vi "Get Strings from Enum__csm.vi"(8 "error in (no error)":errorcluster, 10 "Enum":variant) -> (0 "error out":errorcluster, 1 "String Value":string, 2 "Enum Strings":string[](array[string]), 3 "Enum Name":string)   [LabVIEW 2017, in "API String Arguments Support.lvlib"]
doc: "Returns Enum Strings array, String Value and Enum Name from an Enum."
uses:
  API String Arguments Support.lvlib
  <userlib>/_NEVSTOP/Communicable State Machine(CSM)/Communicable State Machine.lvlib
panel:
  # "[OpenG VI Tags] ***Do Not Remove***"
  # "Get Strings from Enum.vi\n\nReturns Enum Strings array, String Value and Enum Name from an Enum.\n\nPlease visit http://www.OpenG.org to learn about the\nOpen Source LabVIEW software movement.\n\nNOTICE -- YOU MUST LEAVE THIS NOTICE IN PLACE.  PER THE TERMS OF THE LICENSE BELOW, YOU MAY SUBLICENSE THIS SOFTWARE \nIN ANY WAY THAT DOES NOT CONFLICT WITH THIS LICENSE.\n\n### BSD License (http://www.opensource.org/licenses/bsd-license.php) Begin ###\n \nCopyright (c) 2002, Jean-Pierre Drolet <drolet_jp@hotmail.com>\nCopyright (c) 2002-2006, Jim Kring <jim@jimkring.com>\n\nAll rights reserved.\n\nRedistribution and use in source and binary forms, with or without modification, are permitted provided that the following conditions are met:\n\n    * Redistributions of source code must retain the above copyright notice, this list of conditions and the following disclaimer.\n    * Redistributions in binary form must reproduce the above copyright notice, this list of conditions and the following disclaimer in the \n       documentation and/or other materials provided with the distribution.\n    * Neither the name of SciWare, James Kring, Inc., nor the names of its contributors may be used to endorse or promote products derived \n       from this software without specific prior written permission.\n\nTHIS SOFTWARE IS PROVIDED BY THE COPYRIGHT HOLDERS AND CONTRIBUTORS \"AS IS\" AND ANY EXPRESS OR IMPLIED WARRANTIES, \nINCLUDING, BUT NOT LIMITED TO, THE IMPLIED WARRANTIES OF MERCHANTABILITY AND FITNESS FOR A PARTICULAR PURPOSE ARE \nDISCLAIMED. IN NO EVENT SHALL THE COPYRIGHT OWNER OR CONTRIBUTORS BE LIABLE FOR ANY DIRECT, INDIRECT, INCIDENTAL,\n SPECIAL, EXEMPLARY, OR CONSEQUENTIAL DAMAGES (INCLUDING, BUT NOT LIMITED TO, PROCUREMENT OF SUBSTITUTE GOODS OR \nSERVICES; LOSS OF USE, DATA, OR PROFITS; OR BUSINESS INTERRUPTION) HOWEVER CAUSED AND ON ANY THEORY OF LIABILITY, \nWHETHER IN CONTRACT, STRICT LIABILITY, OR TORT (INCLUDING NEGLIGENCE OR OTHERWISE) ARISING IN ANY WAY OUT OF THE USE \nOF THIS SOFTWARE, EVEN IF ADVISED OF THE POSSIBILITY OF SUCH DAMAGE.\n\n### BSD License End ###"
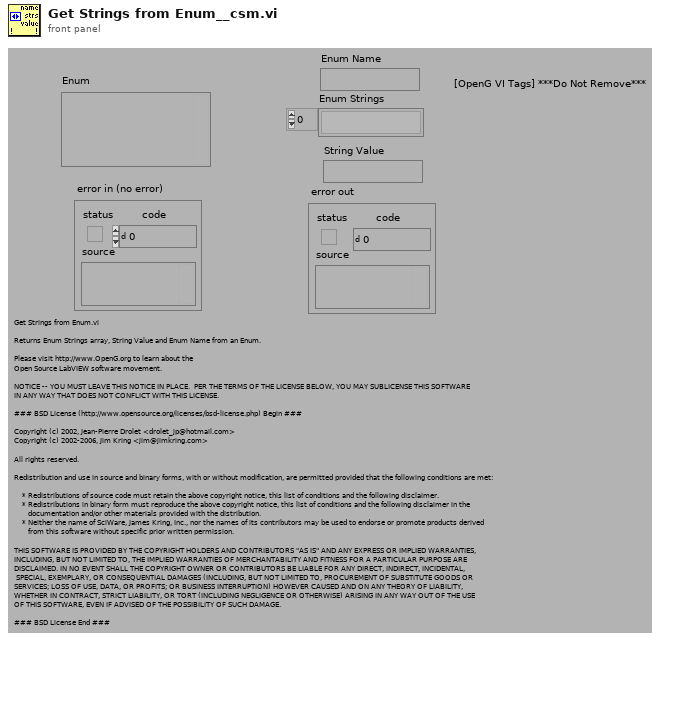
[diagram p1: front panel]
types:
  T1 = cluster{"length":u16, "private":u8, "type":enum8{"<Null>", "I8", "I16", "I32", "I64", "U8", "U16", "U32", "U64", "SGL", "DBL", "EXT", "CSG", "CDB", "CXT", "0x0F", "0x10", "0x11", "0x12", "0x13", "0x14", "Enum U8", "Enum U16", "Enum U32", "Enum U64", "SGL PQ", "DBL PQ", "EXT PQ", "CSG PQ", "CDB PQ", "CXT PQ", "0x1F", "0x20", "Boolean", "0x22", "0x23", "0x24", "0x25", "0x26", "0x27", "0x28", "0x29", "0x2A", "0x2B", "0x2C", "0x2D", "0x2E", "0x2F", "String", "0x31", "Path", "Pict", "0x34", "0x35", "0x36", "DAQ", "0x38", "0x39", "0x3A", "0x3B", "0x3C", "0x3D", "0x3E", "0x3F", "Array", "0x41", "0x42", "0x43", "0x44", "0x45", "0x46", "0x47", "0x48", "0x49", "0x4A", "0x4B", "0x4C", "0x4D", "0x4E", "0x4F", "Cluster", "0x51", "0x52", "Variant", "Waveform", "0x55", "0x56", "0x57", "0x58", "0x59", "0x5A", "0x5B", "0x5C", "0x5D", "0x5E", "Fixed Point", "0x60", "0x61", "0x62", "0x63", "0x64", "0x65", "0x66", "0x67", "0x68", "0x69", "0x6A", "0x6B", "0x6C", "0x6D", "0x6E", "0x6F", "Refnum", "0x71", "0x72", "Set Collection", "Map Collection"}, "# elements":u16}
  T2 = enum8{"<Null>", "I8", "I16", "I32", "I64", "U8", "U16", "U32", "U64", "SGL", "DBL", "EXT", "CSG", "CDB", "CXT", "0x0F", "0x10", "0x11", "0x12", "0x13", "0x14", "Enum U8", "Enum U16", "Enum U32", "Enum U64", "SGL PQ", "DBL PQ", "EXT PQ", "CSG PQ", "CDB PQ", "CXT PQ", "0x1F", "0x20", "Boolean", "0x22", "0x23", "0x24", "0x25", "0x26", "0x27", "0x28", "0x29", "0x2A", "0x2B", "0x2C", "0x2D", "0x2E", "0x2F", "String", "0x31", "Path", "Pict", "0x34", "0x35", "0x36", "DAQ", "0x38", "0x39", "0x3A", "0x3B", "0x3C", "0x3D", "0x3E", "0x3F", "Array", "0x41", "0x42", "0x43", "0x44", "0x45", "0x46", "0x47", "0x48", "0x49", "0x4A", "0x4B", "0x4C", "0x4D", "0x4E", "0x4F", "Cluster", "0x51", "0x52", "Variant", "Waveform", "0x55", "0x56", "0x57", "0x58", "0x59", "0x5A", "0x5B", "0x5C", "0x5D", "0x5E", "Fixed Point", "0x60", "0x61", "0x62", "0x63", "0x64", "0x65", "0x66", "0x67", "0x68", "0x69", "0x6A", "0x6B", "0x6C", "0x6D", "0x6E", "0x6F", "Refnum", "0x71", "0x72", "Set Collection", "Map Collection"}
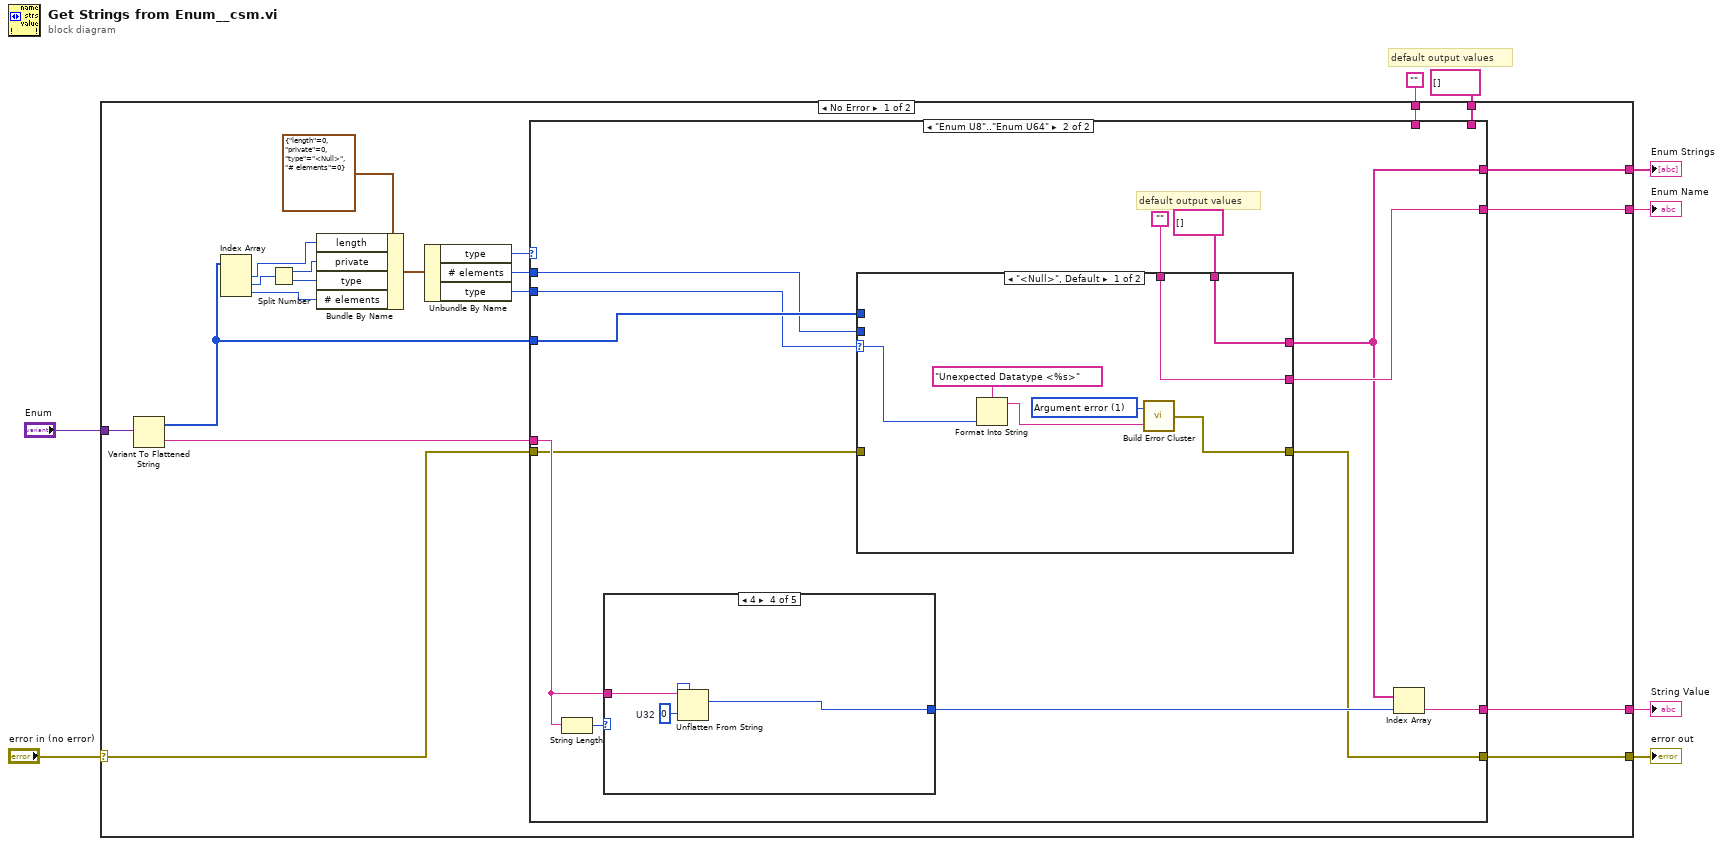
[diagram p0: block diagram]
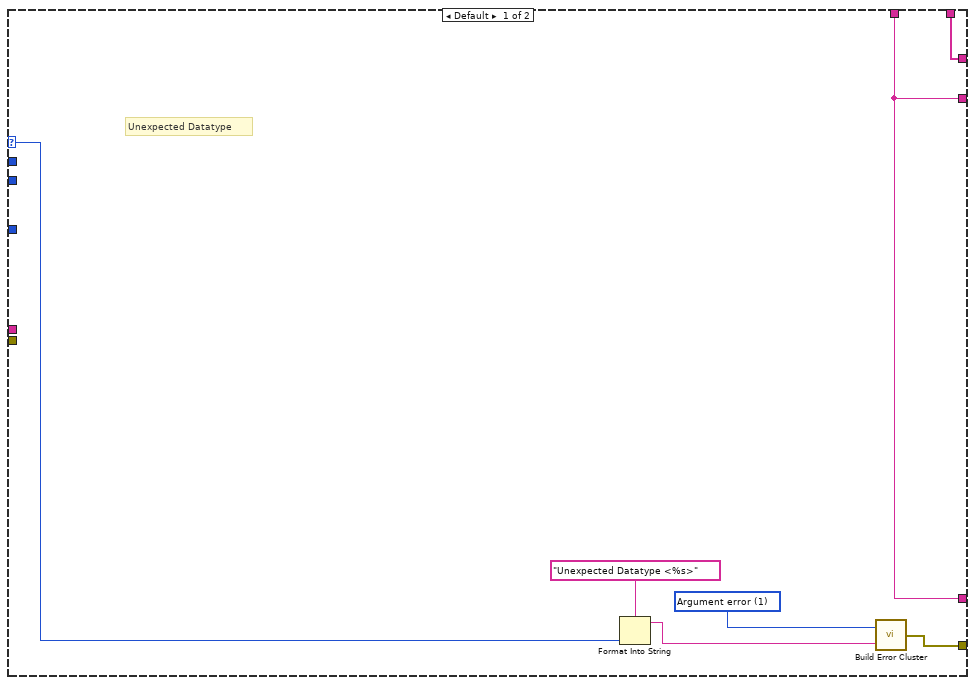
[diagram p2: hidden frame]
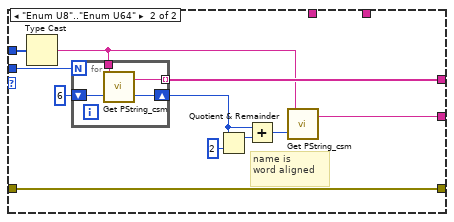
[diagram p3: hidden frame]
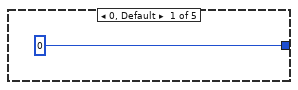
[diagram p4: hidden frame]
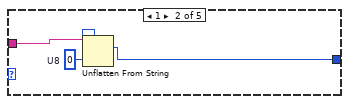
[diagram p5: hidden frame]
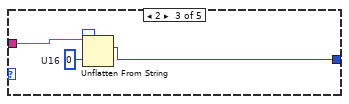
[diagram p6: hidden frame]
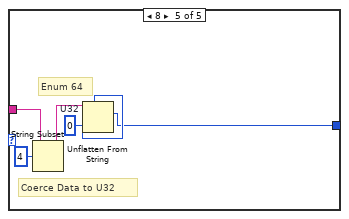
[diagram p7: hidden frame]
diagram:
  # "default output values"
  n1 = case shown="No Error" "error in (no error)" {
    selector: "error in (no error)" -> [w20 w88]
    tunnel: [w28 w88] -> w8
    tunnel: [w23 w87] -> w6
    tunnel: [w22 w86] -> w5
    tunnel: [w21 w86] -> w4
    tunnel: string[] [] -> [w19 w87]
    tunnel: "" -> [w18 w86]
    tunnel: "Enum" -> [w11 _]
    frame No Error {
      n2 = Variant To Flattened String(Variant=w11) -> (data string=w24:string, 1:w25:i16[])
      n3 = Index Array(array=w25) -> (element #1=w13:i16, element #2=w16:i16, element #3=w17:i16)  [unwired: 3 in]
      n4 = Split Number(x=w16) -> (hi(x)=w14:u8, lo(x)=w15:u8)
      n5 = Bundle By Name(cluster=T1 {"length"=0, "private"=0, "type"=enum."<Null>", "# elements"=0} ("Type Descriptor Header"), "length"=w13, "private"=w14, "type"=w15, "# elements"=w17) -> (w27:T1)
      n6 = Unbundle By Name(w27) -> ("type"=w26:T2, "# elements"=w9:u16, "type"=w10:T2)
      n7 = case shown="\"Enum U8\"..\"Enum U64\"" w26 {
        selector: w26 -> [w34 _]
        tunnel: [w31 w41] -> w28
        tunnel: w25 -> [_ w43]
        tunnel: w24 -> [_ w47]
        tunnel: [w30 w40] -> w23
        tunnel: [w29 w44] -> w22
        tunnel: [w29 w45] -> w21
        tunnel: w20 -> [_ w42]
        tunnel: w19 -> [w30 _]
        tunnel: w18 -> [w29 _]
        tunnel: w10 -> [_ w37]
        tunnel: w9 -> [_ w36]
        frame Default {
          w35 = 1 items=["No error", "Argument error", "Memory is full", "Out of zone", "End of file", "File already open", "Generic file I/O error", "File not found", "File permission error", "Disk is full", "Duplicate path", "Too many files open", "System feature not enabled", "Resource file not found", "Cannot add resource", "Resource not found", "Image not found", "Image memory error", "Pen does not exist", "Config type invalid", "Config token not found", "Config parse error", "Config memory error", "Bad external code format", "Bad external code offset", "External code not present", "Null window", "Destroy window error", "Null menu", "Print aborted", "Bad print record", "Print driver error", "Windows error during printing", "Memory error during printing", "Print dialog error", "Generic print error", "Invalid device refnum", "Device not found", "Device parameter error", "Device unit error", "Cannot open device", "Device call aborted", "Generic error", "Cancelled by user", "Object ID too low", "Object ID too high", "Object not in heap", "Unknown heap", "Unknown object (invalid DefProc)", "Unknown object (DefProc not in table)", "Message out of range", "Invalid (null) method", "Unknown message", "Manager call not supported", "Bad address", "Network operation in progress", "Network operation timed out", "Connection is busy", "Network attribute not supported", "Network error", "Address in use", "System out of memory", "Connection aborted", "Connection refused", "Not connected", "Already connected", "Connection closed", "Initialization error (interapplication manager)", "Bad occurrence", "Wait on unbound occurrence handler", "Occurrence queue overflow", "Datalog type conflict", "Unused", "Unrecognized type (interapplication manager)", "Memory corrupt", "Failed to make temporary DLL", "Old CIN version", "Drag socket not found", "Failed to load drop-object", "Failed to register OLE object", "Failed to release OLE object", "Format specifier type mismatch", "Unknown format specifier", "Too few format specifiers", "Too many format specifiers", "Scan failed", "Newer CIN version", "Error converting to variant", "Runtime menu error", "Password tampered", "Variant attribute not found", "Incompatible variant data type", "Event data is not available", "Event Store is not present", "Occurrence is not found", "Event Queue is not created", "Event info is not available", "Refnum passed is NULL", "Error retrieving Class GUID", "Error retrieving CoClass GUID", "Error retrieving TypeLib GUID.", "Bad built application magic bytes.", "Specific driver is different from the specific driver associated with the Logical Name.", "There is no session opened to the class driver.", "Max Error", "MAX - Error with config objects", "MAX - Error loading configuration", "MAX - Group not supported"]
          # "Unexpected Datatype"
          n8 = Format Into String(format string="Unexpected Datatype <%s>" ("Format String"), w34) -> (resulting string=w32:string)  [unwired: 2 in, 1 out]
          n9 = call <userlib>:"Build Error Cluster.vi"("String to Prepend to source (\"\")"=w32, "code"=w35) -> ("error out"=w31:errorcluster)
        }
        frame "Enum U8".."Enum U64" {
          # "default output values"
          n10 = String Length(string=w47) -> (length=w48:i32)
          n11 = case shown="4" w48 {
            tunnel: w47 -> [_ w74 w77 w80 w81]
            tunnel: [u32 0 ("U32") w72 w75 w78 w84] -> w46
            frame 0, Default {
            }
            frame 1 {
              w73 = u8 0  # U8
              n12 = Unflatten From String(type=w73, binary string=w74) -> (value=w72:u8)  [unwired: 3 in, 2 out]
            }
            frame 2 {
              w76 = u16 0  # U16
              n13 = Unflatten From String(type=w76, binary string=w77) -> (value=w75:u16)  [unwired: 3 in, 2 out]
            }
            frame 4 {
              w79 = u32 0  # U32
              n14 = Unflatten From String(type=w79, binary string=w80) -> (value=w78:u32)  [unwired: 3 in, 2 out]
            }
            frame 8 {
              w85 = u32 0  # U32
              # "Coerce Data to U32"
              # "Enum 64"
              n15 = String Subset(string=w81, offset (0)=4) -> (substring=w82:string)  [unwired: 1 in]
              n16 = Unflatten From String(type=w85, binary string=w82) -> (value=w84:u32)  [unwired: 3 in, 2 out]
            }
          }
          n17 = case shown="\"<Null>\", Default" w37 {
            selector: w37 -> [w50 _]
            tunnel: w36 -> [_ w66]
            tunnel: w43 -> [_ w65]
            tunnel: [w55 w64] -> w40
            tunnel: [w54 w63] -> w44
            tunnel: string[] [] -> [w55 _]
            tunnel: "" ("PString") -> [w54 _]
            tunnel: [w49 w56] -> w41
            tunnel: w42 -> [_ w56]
            frame "<Null>", Default {
              w53 = 1 items=["No error", "Argument error", "Memory is full", "Out of zone", "End of file", "File already open", "Generic file I/O error", "File not found", "File permission error", "Disk is full", "Duplicate path", "Too many files open", "System feature not enabled", "Resource file not found", "Cannot add resource", "Resource not found", "Image not found", "Image memory error", "Pen does not exist", "Config type invalid", "Config token not found", "Config parse error", "Config memory error", "Bad external code format", "Bad external code offset", "External code not present", "Null window", "Destroy window error", "Null menu", "Print aborted", "Bad print record", "Print driver error", "Windows error during printing", "Memory error during printing", "Print dialog error", "Generic print error", "Invalid device refnum", "Device not found", "Device parameter error", "Device unit error", "Cannot open device", "Device call aborted", "Generic error", "Cancelled by user", "Object ID too low", "Object ID too high", "Object not in heap", "Unknown heap", "Unknown object (invalid DefProc)", "Unknown object (DefProc not in table)", "Message out of range", "Invalid (null) method", "Unknown message", "Manager call not supported", "Bad address", "Network operation in progress", "Network operation timed out", "Connection is busy", "Network attribute not supported", "Network error", "Address in use", "System out of memory", "Connection aborted", "Connection refused", "Not connected", "Already connected", "Connection closed", "Initialization error (interapplication manager)", "Bad occurrence", "Wait on unbound occurrence handler", "Occurrence queue overflow", "Datalog type conflict", "Unused", "Unrecognized type (interapplication manager)", "Memory corrupt", "Failed to make temporary DLL", "Old CIN version", "Drag socket not found", "Failed to load drop-object", "Failed to register OLE object", "Failed to release OLE object", "Format specifier type mismatch", "Unknown format specifier", "Too few format specifiers", "Too many format specifiers", "Scan failed", "Newer CIN version", "Error converting to variant", "Runtime menu error", "Password tampered", "Variant attribute not found", "Incompatible variant data type", "Event data is not available", "Event Store is not present", "Occurrence is not found", "Event Queue is not created", "Event info is not available", "Refnum passed is NULL", "Error retrieving Class GUID", "Error retrieving CoClass GUID", "Error retrieving TypeLib GUID.", "Bad built application magic bytes.", "Specific driver is different from the specific driver associated with the Logical Name.", "There is no session opened to the class driver.", "Max Error", "MAX - Error with config objects", "MAX - Error loading configuration", "MAX - Group not supported"]
              n18 = Format Into String(format string="Unexpected Datatype <%s>" ("Format String"), w50) -> (resulting string=w51:string)  [unwired: 2 in, 1 out]
              n19 = call <userlib>:"Build Error Cluster.vi"("String to Prepend to source (\"\")"=w51, "code"=w53) -> ("error out"=w49:errorcluster)
            }
            frame "Enum U8".."Enum U64" {
              # "name is\nword aligned"
              n20 = Type Cast(x=w65) -> (*(type *) &x=w61:string)  [unwired: 1 in]
              n21 = for {
                N: w66 -> [_]
                tunnel: w61 -> [w67]
                shift-right: [w68] -> w60
                shift-left: 6 -> [w69]
                tunnel: [w70] -> w64 mode=indexing
                n22 = call <userlib>:"Get PString_csm.vi"("offset (0)"=w69, "String"=w67) -> ("offset past PString"=w68:i32, "PString"=w70:string)
              }
              n23 = Quotient & Remainder(x=w60, y=2) -> (x-y*floor(x/y)=w59:i32)  [unwired: 1 out]
              n24 = Add(x=w60, y=w59) -> (x+y=w62:i32)
              n25 = call <userlib>:"Get PString_csm.vi"("offset (0)"=w62, "String"=w61) -> ("PString"=w63:string)  [unwired: 1 out]
            }
          }
          n26 = Index Array(array=w40, index=w46) -> (element=w45:string)
        }
      }
    }
    frame Error {
    }
  }
  "error out" <- w8
  "Enum Strings" <- w6
  "Enum Name" <- w5
  "String Value" <- w4
